vi "OscTest.vi"(7 "FrequencyCounter":refnum<visa-resource-name>, 8 "error in":errorcluster, 9 "connection information":path, 10 "System Number":string, 11 "Arduino":refnum<visa-resource-name>) -> (0 "error out":errorcluster, 3 "Arduino out":refnum<visa-resource-name>)   [LabVIEW 2024]
uses:
  <vilib>/addons/database/Connection.llb/DB Tools Open Connec (Path).vi
  Agilent 532XX Series/Public/Configure/Measurement/Configure Measurement (Frequency).vi
  <vilib>/addons/database/_DB Variant To Data/Database Variant To Data.xnode
  <vilib>/addons/database/NI_Database_API.lvlib
  Agilent 532XX Series/Agilent 532XX Series.lvlib
panel:
  out "Work Order":string
  out "Unit_Number":string
  out "VoltageSupply":dbl format="%.4f"
  out "Nominal Frequency":string
  out "IsSine":bool=TRUE
  out "TimeStart":string
  in  "DC_SN":string
  out "OscData":string
  out "VcLower":string
  out "VcLower-Frequency":dbl format="%.6f"
  out "Lower Deviation":dbl
  out "VcUpper":string
  out "VcUpper-Frequency":dbl format="%.6f"
  out "Upper Deviation":dbl
  out "VcMiddle-Frequency":dbl format="%.6f"
  out "Symmetry":dbl format="%.6f"
  out "State \"1\"":dbl format="%.6f"
  out "State \"0\"":dbl format="%.6f"
  out "Middle Deviation":dbl
  out "RiseTime":dbl format="%.6f"
  out "FallTime":dbl format="%.6f"
  out "Vpp":dbl format="%.6f"
  out "VcMiddle":string
  out "CurrentSupply":dbl format="%.4f"
  out "OscVoltage":string
types:
  T1 = typedef "NI_Database_API.lvlib/Conn ObjectReference.ctl" = refnum<k1>
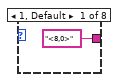
[diagram p3: hidden frame]
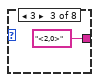
[diagram p4: hidden frame]
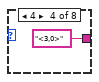
[diagram p5: hidden frame]
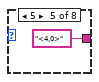
[diagram p6: hidden frame]
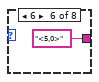
[diagram p7: hidden frame]
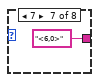
[diagram p8: hidden frame]
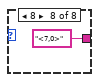
[diagram p9: hidden frame]
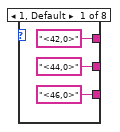
[diagram p10: hidden frame]
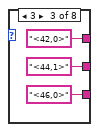
[diagram p11: hidden frame]
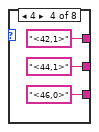
[diagram p12: hidden frame]
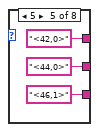
[diagram p13: hidden frame]
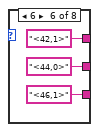
[diagram p14: hidden frame]
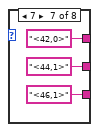
[diagram p15: hidden frame]
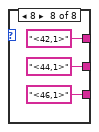
[diagram p16: hidden frame]
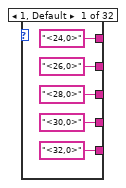
[diagram p17: hidden frame]
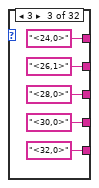
[diagram p18: hidden frame]
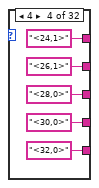
[diagram p19: hidden frame]
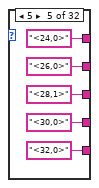
[diagram p20: hidden frame]
diagram:
  n1 = flat-sequence {
    tunnel: [w15] -> w1
    tunnel: w1 -> [w16]
    tunnel: [w23] -> w7
    tunnel: [w24] -> w6
    tunnel: w7 -> [w29]
    tunnel: w6 -> [w28]
    tunnel: [w27] -> w5
    tunnel: [w26] -> w4
    tunnel: [w862] -> w2
    tunnel: w5 -> [w862]
    tunnel: [w861] -> w3
    tunnel: w4 -> [w861]
    frame #0 {
      n2 = Get Date/Time In Seconds() -> (seconds since 1Jan1904=w14:timestamp)
      n3 = Bundle(0, 6) -> (w15:cluster{i32, i32})  [unwired: 1 in]
      n4 = Format Date/Time String(time format string (%c)="%m/%d/%Y %I:%M %p", seconds (now)=w14) -> (date/time string=→"TimeStart":string)  [unwired: 1 in]
      n5 = call "Set Temperature and Rise Time.vi"("Slew Time String"="0", "Temperature String"="25", "Device"=w15) -> ()  [unwired: 3 in, 1 out]
    }
    frame #1 {
      n6 = while {
        tunnel: w16 -> [w22]
        stop <- w18 stop-if-true
        n7 = call "Read Saunders Temperature.vi"("Device"=w22) -> ("Temperature"=w21:dbl)  [unwired: 3 in, 1 out]
        n8 = Wait (ms)(milliseconds to wait=u32 1000) -> ()  [unwired: 1 out]
        n9 = In Range and Coerce(upper limit=26.0, x=w21, lower limit=24.0) -> (In Range?=w18:bool)  [unwired: 1 out]
      }
    }
    frame #2 {
      n10 = local read "Arduino"() -> (w23:refnum<visa-resource-name>)
      n11 = local read "error in"() -> (w24:errorcluster)
      n12 = Wait (ms)(milliseconds to wait=u32 500) -> ()  [unwired: 1 out]
    }
    frame #3 {
      n13 = for {
        N: 32 -> [_]
        shift-right: [w32] -> w27
        shift-left: w29 -> [w34]
        shift-right: [w31] -> w26
        shift-left: w28 -> [w33]
        i -> [w35]
        n14 = for {
          N: 8 -> [_]
          tunnel: w35 -> [w47]
          shift-right: [w44] -> w32
          shift-left: w34 -> [w46]
          shift-right: [w43] -> w31
          shift-left: w33 -> [w45]
          i -> [w49]
          n15 = Increment(x=w49) -> (x+1=w48:i32)
          n16 = flat-sequence {
            tunnel: [w53] -> w42
            tunnel: [w84] -> w41
            tunnel: [w83] -> w40
            tunnel: [w82] -> w39
            tunnel: w48 -> [w53]
            tunnel: w47 -> [w50]
            tunnel: w46 -> [w83]
            tunnel: w45 -> [w80]
            tunnel: [w52] -> w38
            tunnel: [w51] -> w37
            tunnel: w42 -> [w137]
            tunnel: w41 -> [w136]
            tunnel: w40 -> [w135]
            tunnel: w39 -> [w134]
            tunnel: [w133] -> w44
            tunnel: [w132] -> w43
            tunnel: w38 -> [w131]
            tunnel: w37 -> [w130]
            frame #0 {
              n17 = local read "System Number"() -> (w68:string)
              n18 = local write "DC_SN"("" ("DC.SN")) -> ()
              n19 = local read "connection information"() -> (w54:path)
              n20 = Number To Decimal String(number=w53) -> (decimal integer string=w69:string)  [unwired: 1 in]
              n21 = Concatenate Strings("WHERE System=" ("SQL Query"), w68, " AND Rack=", w69, ";" ("string")) -> (w55:string)
              n22 = call-poly <vilib>:"DB Tools Open Connection.vi"("connection information"=w54) -> ("error out"=w65:errorcluster, "connection reference"=w66:T1)  [unwired: 7 in]
              n23 = Increment(x=w50) -> (x+1=w84:i32)
              n24 = call <vilib>:"DB Tools Select Data.vi"("condition"=w55, "error in (no error)"=w65, "columns"=string[] ["Position"], "table"="ACTIVE", "connection reference"=w66) -> ("error out"=w62:errorcluster, "data"=w60:variant[][], "connection reference out"=w64:T1)  [unwired: 1 in]
              n25 = xnode "Database Variant To Data"("database variant"=w60, "error in (no error)"=w62, "type"=string[][] [] ("DC.SN")) -> ("data"=w59:string[][], "error out"=w63:errorcluster)
              n26 = call <vilib>:"DB Tools Close Connection.vi"("error in (no error)"=w63, "connection reference"=w64) -> ("error out"=w56:errorcluster)  [unwired: 5 in]
              n27 = Index Array(array=w59, index (row)=0 ("disabled index (row)"), index (col)=0 ("disabled index (col)")) -> (element=w79:string)
              n28 = Unbundle By Name(w56) -> ("status"=w67:bool)
              n29 = call <vilib>:"Delimited String to 1D String Array.vi"("delimiter"=",", "delimited string"=w79) -> ("string array"=w76:string[])  [unwired: 9 in]
              n30 = Not(x=w67) -> (.not. x?=w52:bool)
              n31 = Index Array(array=w76, index=w50) -> (element=w75:string)
              n32 = call <vilib>:"Clear Errors.vi"("error in (no error)"=w80) -> ("error out"=w82:errorcluster)  [unwired: 5 in, 1 out]
              n33 = Equal?(x="1", y=w75) -> (x = y?=w51:bool)
            }
            frame #1 {
              n34 = And(x=w130, y=w131) -> (x .and. y?=w129:bool)
              n35 = case shown="True" w129 {
                tunnel: w136 -> [_ w183]
                tunnel: w137 -> [_ w182]
                tunnel: w135 -> [w138 w172]
                tunnel: w134 -> [w139 w173]
                tunnel: [w138 w160] -> w133
                tunnel: [w139 w159] -> w132
                frame False {
                }
                frame True {
                  n36 = flat-sequence {
                    tunnel: w182 -> [w189]
                    tunnel: w183 -> [w190]
                    tunnel: [w190] -> w180
                    tunnel: [w189] -> w178
                    tunnel: [w184] -> w142
                    tunnel: w180 -> [w394]
                    tunnel: [w394] -> w179
                    tunnel: w178 -> [w393]
                    tunnel: [w393] -> w177
                    tunnel: [w391] -> w143
                    tunnel: w142 -> [w391]
                    tunnel: [w400] -> w175
                    tunnel: w179 -> [w397]
                    tunnel: w177 -> [w400]
                    tunnel: [w438] -> w144
                    tunnel: w143 -> [w438]
                    tunnel: [w395] -> w141
                    tunnel: w175 -> [w486]
                    tunnel: [w486] -> w174
                    tunnel: [w484] -> w145
                    tunnel: w144 -> [w484]
                    tunnel: w141 -> [w483]
                    tunnel: [w483] -> w140
                    tunnel: w174 -> [w493]
                    tunnel: [w493] -> w176
                    tunnel: w173 -> [w492]
                    tunnel: w172 -> [w491]
                    tunnel: [w489] -> w170
                    tunnel: [w490] -> w169
                    tunnel: w145 -> [w488]
                    tunnel: w140 -> [w487]
                    tunnel: w176 -> [w501]
                    tunnel: [w501] -> w181
                    tunnel: w181 -> [w512]
                    tunnel: [w512] -> w168
                    tunnel: [w503] -> w165
                    tunnel: w168 -> [w515]
                    tunnel: [w515] -> w167
                    tunnel: [w513] -> w166
                    tunnel: w165 -> [w513]
                    tunnel: w167 -> [w516]
                    tunnel: [w516] -> w171
                    tunnel: w166 -> [w520]
                    tunnel: [w517] -> w162
                    tunnel: [w526] -> w164
                    tunnel: w171 -> [w526]
                    tunnel: [w524] -> w163
                    tunnel: w162 -> [w524]
                    tunnel: w164 -> [w537]
                    tunnel: [w537] -> w161
                    tunnel: w163 -> [w530]
                    tunnel: [w540] -> w158
                    tunnel: w161 -> [w539]
                    tunnel: [w539] -> w153
                    tunnel: w170 -> [w555]
                    tunnel: w169 -> [w554]
                    tunnel: [w553] -> w152
                    tunnel: [w552] -> w150
                    tunnel: w158 -> [w551]
                    tunnel: [w550] -> w154
                    tunnel: w153 -> [w550]
                    tunnel: [w556] -> w155
                    tunnel: w154 -> [w556]
                    tunnel: [w558] -> w156
                    tunnel: w155 -> [w558]
                    tunnel: [w574] -> w157
                    tunnel: w156 -> [w574]
                    tunnel: w157 -> [w576]
                    tunnel: w152 -> [w580]
                    tunnel: [w579] -> w151
                    tunnel: w150 -> [w578]
                    tunnel: [w577] -> w149
                    tunnel: [w576] -> w146
                    tunnel: [w840] -> w147
                    tunnel: w146 -> [w840]
                    tunnel: [w843] -> w148
                    tunnel: w147 -> [w843]
                    tunnel: w149 -> [w851]
                    tunnel: [w850] -> w160
                    tunnel: w151 -> [w849]
                    tunnel: [w848] -> w159
                    tunnel: w148 -> [w845]
                    frame #0 {
                      n37 = case shown="2" w189 {
                        tunnel: ["<8,0>" ("string") "<9,0>" ("string") "<2,0>" ("string") "<3,0>" ("string") "<4,0>" ("string") "<5,0>" ("string") "<6,0>" ("string") "<7,0>" ("string")] -> w188
                        frame 1, Default {
                        }
                        frame 2 {
                        }
                        frame 3 {
                        }
                        frame 4 {
                        }
                        frame 5 {
                        }
                        frame 6 {
                        }
                        frame 7 {
                        }
                        frame 8 {
                        }
                      }
                      n38 = case shown="2" w189 {
                        tunnel: ["<42,0>" ("string") "<42,1>" ("string") "<42,0>" ("string") "<42,1>" ("string") "<42,0>" ("string") "<42,1>" ("string") "<42,0>" ("string") "<42,1>" ("string")] -> w193
                        tunnel: ["<44,0>" ("string") "<44,0>" ("string") "<44,1>" ("string") "<44,1>" ("string") "<44,0>" ("string") "<44,0>" ("string") "<44,1>" ("string") "<44,1>" ("string")] -> w192
                        tunnel: ["<46,0>" ("string") "<46,0>" ("string") "<46,0>" ("string") "<46,0>" ("string") "<46,1>" ("string") "<46,1>" ("string") "<46,1>" ("string") "<46,1>" ("string")] -> w191
                        frame 1, Default {
                        }
                        frame 2 {
                        }
                        frame 3 {
                        }
                        frame 4 {
                        }
                        frame 5 {
                        }
                        frame 6 {
                        }
                        frame 7 {
                        }
                        frame 8 {
                        }
                      }
                      n39 = case shown="2" w190 {
                        tunnel: ["<32,0>" ("string") "<32,0>" ("string") "<32,0>" ("string") "<32,0>" ("string") "<32,0>" ("string") "<32,0>" ("string") "<32,0>" ("string") "<32,0>" ("string") "<32,0>" ("string") "<32,0>" ("string") "<32,0>" ("string") "<32,0>" ("string") "<32,0>" ("string") "<32,0>" ("string") "<32,0>" ("string") "<32,0>" ("string") "<32,1>" ("string") "<32,1>" ("string") "<32,1>" ("string") "<32,1>" ("string") "<32,1>" ("string") "<32,1>" ("string") "<32,1>" ("string") "<32,1>" ("string") "<32,1>" ("string") "<32,1>" ("string") "<32,1>" ("string") "<32,1>" ("string") "<32,1>" ("string") "<32,1>" ("string") "<32,1>" ("string") "<32,1>" ("string")] -> w194
                        tunnel: ["<30,0>" ("string") "<30,0>" ("string") "<30,0>" ("string") "<30,0>" ("string") "<30,0>" ("string") "<30,0>" ("string") "<30,0>" ("string") "<30,0>" ("string") "<30,1>" ("string") "<30,1>" ("string") "<30,1>" ("string") "<30,1>" ("string") "<30,1>" ("string") "<30,1>" ("string") "<30,1>" ("string") "<30,1>" ("string") "<30,0>" ("string") "<30,0>" ("string") "<30,0>" ("string") "<30,0>" ("string") "<30,0>" ("string") "<30,0>" ("string") "<30,0>" ("string") "<30,0>" ("string") "<30,1>" ("string") "<30,1>" ("string") "<30,1>" ("string") "<30,1>" ("string") "<30,1>" ("string") "<30,1>" ("string") "<30,1>" ("string") "<30,1>" ("string")] -> w195
                        tunnel: ["<28,0>" ("string") "<28,0>" ("string") "<28,0>" ("string") "<28,0>" ("string") "<28,1>" ("string") "<28,1>" ("string") "<28,1>" ("string") "<28,1>" ("string") "<28,0>" ("string") "<28,0>" ("string") "<28,0>" ("string") "<28,0>" ("string") "<28,1>" ("string") "<28,1>" ("string") "<28,1>" ("string") "<28,1>" ("string") "<28,0>" ("string") "<28,0>" ("string") "<28,0>" ("string") "<28,0>" ("string") "<28,1>" ("string") "<28,1>" ("string") "<28,1>" ("string") "<28,1>" ("string") "<28,0>" ("string") "<28,0>" ("string") "<28,0>" ("string") "<28,0>" ("string") "<28,1>" ("string") "<28,1>" ("string") "<28,1>" ("string") "<28,1>" ("string")] -> w196
                        tunnel: ["<26,0>" ("string") "<26,0>" ("string") "<26,1>" ("string") "<26,1>" ("string") "<26,0>" ("string") "<26,0>" ("string") "<26,1>" ("string") "<26,1>" ("string") "<26,0>" ("string") "<26,0>" ("string") "<26,1>" ("string") "<26,1>" ("string") "<26,0>" ("string") "<26,0>" ("string") "<26,1>" ("string") "<26,1>" ("string") "<26,0>" ("string") "<26,0>" ("string") "<26,1>" ("string") "<26,1>" ("string") "<26,0>" ("string") "<26,0>" ("string") "<26,1>" ("string") "<26,1>" ("string") "<26,0>" ("string") "<26,0>" ("string") "<26,1>" ("string") "<26,1>" ("string") "<26,0>" ("string") "<26,0>" ("string") "<26,1>" ("string") "<26,1>" ("string")] -> w197
                        tunnel: ["<24,0>" ("string") "<24,1>" ("string") "<24,0>" ("string") "<24,1>" ("string") "<24,0>" ("string") "<24,1>" ("string") "<24,0>" ("string") "<24,1>" ("string") "<24,0>" ("string") "<24,1>" ("string") "<24,0>" ("string") "<24,1>" ("string") "<24,0>" ("string") "<24,1>" ("string") "<24,0>" ("string") "<24,1>" ("string") "<24,0>" ("string") "<24,1>" ("string") "<24,0>" ("string") "<24,1>" ("string") "<24,0>" ("string") "<24,1>" ("string") "<24,0>" ("string") "<24,1>" ("string") "<24,0>" ("string") "<24,1>" ("string") "<24,0>" ("string") "<24,1>" ("string") "<24,0>" ("string") "<24,1>" ("string") "<24,0>" ("string") "<24,1>" ("string")] -> w198
                        frame 1, Default {
                        }
                        frame 2 {
                        }
                        frame 3 {
                        }
                        frame 4 {
                        }
                        frame 5 {
                        }
                        frame 6 {
                        }
                        frame 7 {
                        }
                        frame 8 {
                        }
                        frame 9 {
                        }
                        frame 10 {
                        }
                        frame 11 {
                        }
                        frame 12 {
                        }
                        frame 13 {
                        }
                        frame 14 {
                        }
                        frame 15 {
                        }
                        frame 16 {
                        }
                        frame 17 {
                        }
                        frame 18 {
                        }
                        frame 19 {
                        }
                        frame 20 {
                        }
                        frame 21 {
                        }
                        frame 22 {
                        }
                        frame 23 {
                        }
                        frame 24 {
                        }
                        frame 25 {
                        }
                        frame 26 {
                        }
                        frame 27 {
                        }
                        frame 28 {
                        }
                        frame 29 {
                        }
                        frame 30 {
                        }
                        frame 31 {
                        }
                        frame 32 {
                        }
                      }
                      n40 = Build Array(w188, w193, w192, w191, w198, w197, w196, w195, w194, "<48,0>" ("string"), "<50,0>" ("string"), "<52,0>" ("string")) -> (w184:string[])
                    }
                    frame #1 {
                      n41 = Wait (ms)(milliseconds to wait=u32 500) -> ()  [unwired: 1 out]
                    }
                    frame #2 {
                      # "Gets the latest TimeStart from this System/Rack/Position meaning it will be associated with the oscillator that is currently in the spot"
                      # "Data Grabbed:\nIsSine:\n-Boolean that identifies if the Waveform is equal to sine to ensure the frequency counter can be set up for the correct wave\nOscVoltage:\n-The amount of voltage that the oscillator receives as input\nGate Time \n-The period over which the counter accumulates the number of input signal cycles\nNominal Frequency\n- Reference value or a standard against which other frequencies are measured or compared\nDC_SN\n-Unique date code/serial number that identifies the device that is being tested"
                      # "Gets the latest TimeStart from this System/Rack/Position meaning it will be associated with the oscillator that is currently in the spot"
                      n42 = local read "connection information"() -> (w407:path)
                      n43 = local read "System Number"() -> (w437:string)
                      n44 = Number To Decimal String(number=w400) -> (decimal integer string=w403:string)  [unwired: 1 in]
                      n45 = Number To Decimal String(number=w397) -> (decimal integer string=w396:string)  [unwired: 1 in]
                      n46 = Concatenate Strings("WHERE SystemNumber=" ("SQL Query"), w437, "AND RackNumber=" ("string"), w403, "AND PositionNumber=" ("string"), w396, "ORDER BY TimeStart DESC" ("string")) -> (w406:string)
                      n47 = call-poly <vilib>:"DB Tools Open Connection.vi"("connection information"=w407) -> ("error out"=w414:errorcluster, "connection reference"=w415:T1)  [unwired: 7 in]
                      n48 = call <vilib>:"DB Tools Select Data.vi"("condition"=w406, "error in (no error)"=w414, "table"="MASTER", "connection reference"=w415) -> ("error out"=w411:errorcluster, "data"=w409:variant[][], "connection reference out"=w413:T1)  [unwired: 2 in]
                      n49 = xnode "Database Variant To Data"("database variant"=w409, "error in (no error)"=w411, "type"=string[][] [] ("DC.SN")) -> ("data"=w405:string[][], "error out"=w412:errorcluster)
                      n50 = call <vilib>:"DB Tools Close Connection.vi"("error in (no error)"=w412, "connection reference"=w413) -> ("error out"=w404:errorcluster)  [unwired: 5 in]
                      n51 = Index Array(array=w405, index (row)=0 ("disabled index (row)")) -> (element=w419:string[])  [unwired: 1 in]
                      n52 = Unbundle By Name(w404) -> ("status"=w424:bool)
                      n53 = Index Array(array=w419, index=8) -> (element=w430:string)
                      n54 = Index Array(array=w419, index=0) -> (element=w429:string)
                      n55 = Index Array(array=w419, index=9) -> (element=→"OscVoltage":string)
                      n56 = Index Array(array=w419, index=1) -> (element=w418:string)
                      n57 = Index Array(array=w419, index=2) -> (element=w416:string)
                      n58 = Index Array(array=w419, index=12) -> (element=w402:string)
                      n59 = Index Array(array=w419, index=10) -> (element=w431:string)
                      n60 = local write "Nominal Frequency"(w430) -> ()
                      n61 = local write "DC_SN"(w429) -> ()
                      n62 = local write "Unit_Number"(w402) -> ()
                      n63 = Concatenate Strings(w418, "-" ("string"), w416) -> (w401:string)
                      n64 = Equal?(x="Sine", y=w431) -> (x = y?=w398:bool)
                      n65 = local write "Work Order"(w401) -> ()
                      n66 = local write "IsSine"(w398) -> ()
                      n67 = Not(x=w424) -> (.not. x?=w395:bool)
                    }
                    frame #3 {
                      n68 = Wait (ms)(milliseconds to wait=u32 500) -> ()  [unwired: 1 out]
                    }
                    frame #4 {
                      n69 = case shown="True" w487 {
                        tunnel: w492 -> [w495 w500]
                        tunnel: w491 -> [w494 w499]
                        tunnel: [w494 w498] -> w490
                        tunnel: [w495 w497] -> w489
                        tunnel: w488 -> [_ w496]
                        frame False {
                        }
                        frame True {
                          n70 = call "Arduino Command Builder.vi"("error in"=w500, "Commands"=w496, "Arduino in"=w499) -> ("error out"=w497:errorcluster, "Arduino out"=w498:refnum<visa-resource-name>)  [unwired: 7 in]
                        }
                      }
                    }
                    frame #5 {
                      n71 = Wait (ms)(milliseconds to wait=u32 1000 ("millisecond multiple")) -> ()  [unwired: 1 out]
                    }
                    frame #6 {
                      w508 = u16 0 items=["channel 1", "channel 2", "channel 3"] ("channel (ch1:0)")
                      # "Sets the current and voltage limits, and ensures they are within a range to prevent anything from blowing up for channel 1"
                      # "Sets the voltage equal to the value of the OscVoltage which is gotten from the part number (channel 1)"
                      n72 = local read "OscVoltage"() -> (w511:string)
                      n73 = Fract/Exp String To Number(string=w511) -> (number=w504:dbl)  [unwired: 3 in, 1 out]
                      n74 = call "Tek PS2520G Configure Supply24.vi"("GPIB #"=u8 0, "voltage limit"=w504, "Address"=u8 8, "channel (ch1:0)"=w508, "current limit"=1.5, "Switch Output"=TRUE, "output (t:on)"=TRUE) -> ("error out"=w503:errorcluster)  [unwired: 1 in]
                    }
                    frame #7 {
                      n75 = Wait (ms)(milliseconds to wait=u32 1000) -> ()  [unwired: 1 out]
                    }
                    frame #8 {
                      w521 = u16 0 items=["channel 1", "channel 2", "channel 3"] ("channel (ch1:0)")
                      n76 = call "Tek PS2520G Check Volt and Current24.vi"("GPIB #"=u8 0, "Address"=u8 8, "channel (ch1:0)"=w521, "error in (no error)"=w520) -> ("actual output voltage"=→"VoltageSupply":dbl, "actual output current"=→"CurrentSupply":dbl, "error out"=w517:errorcluster)  [unwired: 2 in]
                    }
                    frame #9 {
                      n77 = Wait (ms)(milliseconds to wait=u32 1000) -> ()  [unwired: 1 out]
                    }
                    frame #10 {
                      w532 = u16 0 items=["channel 1", "channel 2", "channel 3"] ("channel (ch1:0)")
                      n78 = call "Tek PS2520G Configure Supply24.vi"("GPIB #"=u8 0, "voltage limit"=0.0, "Address"=u8 8, "channel (ch1:0)"=w532, "current limit"=1.5, "error in (no error)"=w530, "Switch Output"=FALSE, "output (t:on)"=FALSE) -> ("error out"=w527:errorcluster)
                      n79 = Unbundle By Name(w527) -> ("status"=w536:bool)
                      n80 = case shown="False" w536 {
                        frame False {
                        }
                        frame True {
                          n81 = VISA Clear(VISA resource name=refnum<visa-resource-name> "GPIB0::8::INSTR") -> ()  [unwired: 1 in, 2 out]
                        }
                      }
                    }
                    frame #11 {
                      n82 = case shown="2" w539 {
                        tunnel: ["<8,1>" ("string") "<9,1>" ("string") "<2,1>" ("string") "<3,1>" ("string") "<4,1>" ("string") "<5,1>" ("string") "<6,1>" ("string") "<7,1>" ("string")] -> w541
                        frame 1, Default {
                        }
                        frame 2 {
                        }
                        frame 3 {
                        }
                        frame 4 {
                        }
                        frame 5 {
                        }
                        frame 6 {
                        }
                        frame 7 {
                        }
                        frame 8 {
                        }
                      }
                      n83 = Build Array(w541) -> (w540:string[])
                    }
                    frame #12 {
                      n84 = call "Arduino Command Builder.vi"("error in"=w555, "Commands"=w551, "Arduino in"=w554) -> ("error out"=w553:errorcluster, "Arduino out"=w552:refnum<visa-resource-name>)  [unwired: 7 in]
                    }
                    frame #13 {
                      n85 = Wait (ms)(milliseconds to wait=u32 500 ("millisecond multiple")) -> ()  [unwired: 1 out]
                    }
                    frame #14 {
                      n86 = disable-structure shown="Enabled" {
                        frame Disabled {
                          # "Setting the Impedance and Coupling for AC or DC"
                          n87 = local read "IsSine"() -> (w559:bool)
                          n88 = case shown="True" w559 {
                            frame False {
                              n89 = flat-sequence {
                                frame #0 {
                                n90 = Send(0:0 ("bus"), 2:i16 3 ("address"), 5:"INP:COUP DC " ("data string")) -> ()  [unwired: 2 in, 3 out]
                                }
                                frame #1 {
                                n91 = Wait (ms)(milliseconds to wait=u32 500 ("millisecond multiple")) -> ()  [unwired: 1 out]
                                }
                                frame #2 {
                                n92 = Send(0:0 ("bus"), 2:i16 3 ("address"), 5:"INP:IMP 1.0E6" ("data string")) -> ()  [unwired: 2 in, 3 out]
                                }
                              }
                            }
                            frame True {
                              n93 = flat-sequence {
                                frame #0 {
                                n94 = Send(0:0 ("bus"), 2:i16 3 ("address"), 5:"INP:COUP AC " ("data string")) -> ()  [unwired: 2 in, 3 out]
                                }
                                frame #1 {
                                n95 = Wait (ms)(milliseconds to wait=u32 500 ("millisecond multiple")) -> ()  [unwired: 1 out]
                                }
                                frame #2 {
                                n96 = Send(0:0 ("bus"), 2:i16 3 ("address"), 5:"INP:IMP 50" ("data string")) -> ()  [unwired: 2 in, 3 out]
                                }
                              }
                            }
                          }
                        }
                        frame Enabled {
                        }
                      }
                    }
                    frame #15 {
                      n97 = Wait (ms)(milliseconds to wait=u32 500 ("millisecond multiple")) -> ()  [unwired: 1 out]
                    }
                    frame #16 {
                      n98 = flat-sequence {
                        tunnel: w576 -> [w621]
                        tunnel: [w619] -> w581
                        tunnel: w581 -> [w634]
                        tunnel: w580 -> [w633]
                        tunnel: [w632] -> w579
                        tunnel: w578 -> [w630]
                        tunnel: [w631] -> w577
                        frame #0 {
                          w582 = 0.0 ("Is")
                          # "Resets all these variables"
                          n99 = local write "State \"0\""(w582) -> ()
                          n100 = local write "FallTime"(w582) -> ()
                          n101 = local write "VcMiddle-Frequency"(w582) -> ()
                          n102 = local write "VcUpper-Frequency"(w582) -> ()
                          n103 = local write "Symmetry"(w582) -> ()
                          n104 = local write "VcLower-Frequency"(w582) -> ()
                          n105 = local write "State \"1\""(w582) -> ()
                          n106 = local write "RiseTime"(w582) -> ()
                        }
                        frame #1 {
                          n107 = Wait (ms)(milliseconds to wait=u32 500 ("millisecond multiple")) -> ()  [unwired: 1 out]
                          n108 = VISA Clear(VISA resource name=refnum<visa-resource-name> "GPIB0::3::INSTR") -> ()  [unwired: 1 in, 2 out]
                        }
                        frame #2 {
                          # "Grabs all the relevant data for the wave at its true voltage and the current that it draws from it"
                          # "Grabs the Frequency and accounts for error values that are out of range based on nominal frequency"
                          n109 = call "Frequency Counter Waveform.vi"("Channel(1,2,3)"=enum16{"Channel 1", "Channel 2", "Channel 3"}."Channel 1", "VISA resource name"=refnum<visa-resource-name> "GPIB0::3::INSTR") -> ("Symmetry"=→"Symmetry":dbl, "Vmax"=w604:dbl, "Vmin"=w605:dbl, "RTime"=w608:dbl, "FTime"=w607:dbl, "error out"=w592:errorcluster)  [unwired: 7 in, 1 out]
                          n110 = Unbundle By Name(w592) -> ("status"=w591:bool)
                          n111 = In Range and Coerce(upper limit=20.0, x=w604, lower limit=-20.0) -> (coerced(x)=w589:dbl)  [unwired: 1 out]
                          n112 = In Range and Coerce(upper limit=20.0, x=w605, lower limit=-20.0) -> (coerced(x)=w587:dbl)  [unwired: 1 out]
                          n113 = In Range and Coerce(upper limit=500.0, x=w608, lower limit=0.0) -> (coerced(x)=→"RiseTime":dbl)  [unwired: 1 out]
                          n114 = In Range and Coerce(upper limit=500.0, x=w607, lower limit=0.0) -> (coerced(x)=→"FallTime":dbl)  [unwired: 1 out]
                          n115 = local read "IsSine"() -> (w590:bool)
                          n116 = case shown="True" w591 {
                            frame False {
                            }
                            frame True {
                              n117 = VISA Clear(VISA resource name=refnum<visa-resource-name> "GPIB0::3::INSTR") -> ()  [unwired: 1 in, 2 out]
                            }
                          }
                          n118 = case shown="True" w590 {
                            tunnel: w589 -> [w615 w617]
                            tunnel: [w611 w617] -> w588
                            tunnel: w587 -> [w614 w616]
                            tunnel: [w610 w616] -> w586
                            frame False {
                              n119 = Divide(x=w615, y=0.185) -> (x/y=w611:dbl)
                              n120 = Divide(x=w614, y=0.185) -> (x/y=w610:dbl)
                            }
                            frame True {
                            }
                          }
                          "State \"1\"" <- w588
                          "State \"0\"" <- w586
                          n121 = Subtract(x=w589, y=w587) -> (x-y=→"Vpp":dbl)
                        }
                        frame #3 {
                          n122 = case shown="1, Default" w621 {
                            tunnel: ["<21,1>" ("string") "<20,1>" ("string") "<19,1>" ("string") "<18,1>" ("string") "<17,1>" ("string") "<16,1>" ("string") "<15,1>" ("string") "<14,1>" ("string")] -> w620
                            frame 1, Default {
                            }
                            frame 2 {
                            }
                            frame 3 {
                            }
                            frame 4 {
                            }
                            frame 5 {
                            }
                            frame 6 {
                            }
                            frame 7 {
                            }
                            frame 8 {
                            }
                          }
                          n123 = Build Array(w620) -> (w619:string[])
                        }
                        frame #4 {
                          n124 = call "Arduino Command Builder.vi"("error in"=w633, "Commands"=w634, "Arduino in"=w630) -> ("error out"=w632:errorcluster, "Arduino out"=w631:refnum<visa-resource-name>)  [unwired: 7 in]
                        }
                        frame #5 {
                          n125 = Wait (ms)(milliseconds to wait=u32 1000) -> ()  [unwired: 1 out]
                        }
                        frame #6 {
                          n126 = flat-sequence {
                            tunnel: [w655] -> w639
                            tunnel: [w662] -> w638
                            tunnel: w639 -> [w662]
                            tunnel: w638 -> [w665]
                            tunnel: [w664] -> w636
                            tunnel: [w676] -> w637
                            frame #0 {
                              w659 = u16 1 items=["channel 1", "channel 2", "channel 3"] ("channel (ch1:0)")
                              n127 = local read "OscVoltage"() -> (w652:string)
                              n128 = Format Value(string ("")=w652, format string="%.2p") -> (output string=w651:string)  [unwired: 1 in]
                              n129 = Fract/Exp String To Number(use system decimal point (T)=TRUE, string=w651, default (0 dbl)=0.0 ("default (0 DBL)")) -> (number=w648:dbl)  [unwired: 1 in, 1 out]
                              n130 = Divide(x=w648, y=2.0) -> (x/y=w647:dbl)
                              n131 = call "Tek PS2520G Configure Supply24.vi"("GPIB #"=u8 0, "voltage limit"=w647, "Address"=u8 8, "channel (ch1:0)"=w659, "current limit"=1.5, "Switch Output"=FALSE, "output (t:on)"=TRUE) -> ("error out"=w655:errorcluster)  [unwired: 1 in]
                            }
                            frame #1 {
                              n132 = Wait (ms)(milliseconds to wait=u32 5000) -> ()  [unwired: 1 out]
                            }
                            frame #2 {
                              w666 = u16 1 items=["channel 1", "channel 2", "channel 3"] ("channel (ch1:0)")
                              n133 = call "Tek PS2520G Check Volt and Current24.vi"("GPIB #"=u8 0, "Address"=u8 8, "channel (ch1:0)"=w666, "error in (no error)"=w665) -> ("actual output voltage"=w670:dbl, "error out"=w669:errorcluster)  [unwired: 2 in, 1 out]
                              n134 = Unbundle By Name(w669) -> ("status"=w671:bool)
                              n135 = Number To Fractional String(number=w670, precision (6)=i16 2) -> (F-format string=w664:string)  [unwired: 2 in]
                              n136 = case shown="False" w671 {
                                frame False {
                                }
                                frame True {
                                n137 = VISA Clear(VISA resource name=refnum<visa-resource-name> "GPIB0::8::INSTR") -> ()  [unwired: 1 in, 2 out]
                                }
                              }
                            }
                            frame #3 {
                              n138 = Wait (ms)(milliseconds to wait=u32 500) -> ()  [unwired: 1 out]
                            }
                            frame #4 {
                              n139 = for {
                                N: 5 -> [_]
                                tunnel: [w677] -> w676
                                stop <- w678 continue-if-true
                                w682 = 1 items=["Channel 1"=1, "Channel 2"=2, "Channel 3"=3] ("Channel (1:Channel 1)")
                                n140 = local read "FrequencyCounter"() -> (w689:refnum<visa-resource-name>)
                                n141 = call "Initialize.vi"("VISA resource name"=w689) -> ("error out"=w684:errorcluster, "VISA resource name out"=w683:refnum<visa-resource-name>)  [unwired: 9 in]
                                n142 = call "Configure Frequency Gate.vi"("error in (no error)"=w684, "Time Resolution (0.1 s)"=0.1 ("number"), "VISA resource name"=w683) -> ("error out"=w693:errorcluster, "VISA resource name out"=w690:refnum<visa-resource-name>)  [unwired: 7 in]
                                n143 = call-poly "Configure Measurement.vi"("error in (no error)"=w693, "Channel (1:Channel 1)"=w682, "VISA resource name"=w690) -> ("error out"=w692:errorcluster, "VISA resource name out"=w691:refnum<visa-resource-name>)  [unwired: 2 in, 5 out]
                                n144 = call "Read Measurement (Single).vi"("error in (no error)"=w692, "VISA resource name"=w691) -> ("error out"=w686:errorcluster, "Measurement"=w687:dbl, "VISA resource name out"=w685:refnum<visa-resource-name>)  [unwired: 7 in]
                                n145 = call "Close.vi"("error in (no error)"=w686, "VISA resource name"=w685) -> ("error out"=w688:errorcluster)  [unwired: 9 in]
                                n146 = In Range and Coerce(upper limit=5000000000.0, x=w687, lower limit=0.0) -> (coerced(x)=w677:dbl)  [unwired: 1 out]
                                n147 = Unbundle By Name(w688) -> ("status"=w678:bool)
                                n148 = case shown="True" w678 {
                                frame False {
                                }
                                frame True {
                                n149 = local read "FrequencyCounter"() -> (w694:refnum<visa-resource-name>)
                                n150 = VISA Clear(VISA resource name=w694) -> ()  [unwired: 1 in, 2 out]
                                }
                                }
                              }
                            }
                          }
                          n151 = local read "Nominal Frequency"() -> (w645:string)
                          n152 = Fract/Exp String To Number(string=w645) -> (number=w646:dbl)  [unwired: 3 in, 1 out]
                          n153 = Multiply(x=w646, y=1000000.0) -> (x*y=w644:dbl)
                          n154 = Subtract(x=w637, y=w644) -> (x-y=w642:dbl)
                          n155 = Absolute Value(x=w642) -> (abs(x)=w641:dbl)
                          n156 = Divide(x=w641, y=w646) -> (x/y=→"Middle Deviation":dbl)
                          "VcMiddle-Frequency" <- w637
                          "VcMiddle" <- w636
                        }
                        frame #7 {
                          n157 = Wait (ms)(milliseconds to wait=u32 1000) -> ()  [unwired: 1 out]
                        }
                        frame #8 {
                          n158 = flat-sequence {
                            tunnel: [w712] -> w701
                            tunnel: [w719] -> w702
                            tunnel: w701 -> [w719]
                            tunnel: w702 -> [w722]
                            tunnel: [w733] -> w704
                            frame #0 {
                              w716 = u16 1 items=["channel 1", "channel 2", "channel 3"] ("channel (ch1:0)")
                              n159 = local read "OscVoltage"() -> (w708:string)
                              n160 = Format Value(string ("")=w708, format string="%.2p") -> (output string=w707:string)  [unwired: 1 in]
                              n161 = Fract/Exp String To Number(use system decimal point (T)=TRUE, string=w707, default (0 dbl)=0.0 ("default (0 DBL)")) -> (number=w711:dbl)  [unwired: 1 in, 1 out]
                              n162 = call "Tek PS2520G Configure Supply24.vi"("GPIB #"=u8 0, "voltage limit"=w711, "Address"=u8 8, "channel (ch1:0)"=w716, "current limit"=1.5, "Switch Output"=FALSE, "output (t:on)"=TRUE) -> ("error out"=w712:errorcluster)  [unwired: 1 in]
                            }
                            frame #1 {
                              n163 = Wait (ms)(milliseconds to wait=u32 5000) -> ()  [unwired: 1 out]
                            }
                            frame #2 {
                              w723 = u16 1 items=["channel 1", "channel 2", "channel 3"] ("channel (ch1:0)")
                              n164 = call "Tek PS2520G Check Volt and Current24.vi"("GPIB #"=u8 0, "Address"=u8 8, "channel (ch1:0)"=w723, "error in (no error)"=w722) -> ("actual output voltage"=w727:dbl, "error out"=w726:errorcluster)  [unwired: 2 in, 1 out]
                              n165 = Unbundle By Name(w726) -> ("status"=w728:bool)
                              n166 = Number To Fractional String(number=w727, precision (6)=i16 2) -> (F-format string=→"VcUpper":string)  [unwired: 2 in]
                              n167 = case shown="True" w728 {
                                frame False {
                                }
                                frame True {
                                n168 = VISA Clear(VISA resource name=refnum<visa-resource-name> "GPIB0::8::INSTR") -> ()  [unwired: 1 in, 2 out]
                                }
                              }
                            }
                            frame #3 {
                              n169 = Wait (ms)(milliseconds to wait=u32 500) -> ()  [unwired: 1 out]
                            }
                            frame #4 {
                              n170 = for {
                                N: 5 -> [_]
                                tunnel: [w734] -> w733
                                stop <- w735 continue-if-true
                                w739 = 1 items=["Channel 1"=1, "Channel 2"=2, "Channel 3"=3] ("Channel (1:Channel 1)")
                                n171 = local read "FrequencyCounter"() -> (w746:refnum<visa-resource-name>)
                                n172 = call "Initialize.vi"("VISA resource name"=w746) -> ("error out"=w741:errorcluster, "VISA resource name out"=w740:refnum<visa-resource-name>)  [unwired: 9 in]
                                n173 = call "Configure Frequency Gate.vi"("error in (no error)"=w741, "Time Resolution (0.1 s)"=0.1 ("number"), "VISA resource name"=w740) -> ("error out"=w750:errorcluster, "VISA resource name out"=w747:refnum<visa-resource-name>)  [unwired: 7 in]
                                n174 = call-poly "Configure Measurement.vi"("error in (no error)"=w750, "Channel (1:Channel 1)"=w739, "VISA resource name"=w747) -> ("error out"=w749:errorcluster, "VISA resource name out"=w748:refnum<visa-resource-name>)  [unwired: 2 in, 5 out]
                                n175 = call "Read Measurement (Single).vi"("error in (no error)"=w749, "VISA resource name"=w748) -> ("error out"=w743:errorcluster, "Measurement"=w744:dbl, "VISA resource name out"=w742:refnum<visa-resource-name>)  [unwired: 7 in]
                                n176 = call "Close.vi"("error in (no error)"=w743, "VISA resource name"=w742) -> ("error out"=w745:errorcluster)  [unwired: 9 in]
                                n177 = In Range and Coerce(upper limit=5000000000.0, x=w744, lower limit=0.0) -> (coerced(x)=w734:dbl)  [unwired: 1 out]
                                n178 = Unbundle By Name(w745) -> ("status"=w735:bool)
                                n179 = case shown="False" w735 {
                                frame False {
                                }
                                frame True {
                                n180 = local read "FrequencyCounter"() -> (w751:refnum<visa-resource-name>)
                                n181 = VISA Clear(VISA resource name=w751) -> ()  [unwired: 1 in, 2 out]
                                }
                                }
                              }
                            }
                          }
                          n182 = local read "Nominal Frequency"() -> (w699:string)
                          n183 = Fract/Exp String To Number(string=w699) -> (number=w698:dbl)  [unwired: 3 in, 1 out]
                          n184 = Multiply(x=w698, y=1000000.0) -> (x*y=w700:dbl)
                          n185 = Subtract(x=w704, y=w700) -> (x-y=w697:dbl)
                          n186 = Absolute Value(x=w697) -> (abs(x)=w696:dbl)
                          n187 = Divide(x=w696, y=w698) -> (x/y=→"Upper Deviation":dbl)
                          "VcUpper-Frequency" <- w704
                        }
                        frame #9 {
                          n188 = Wait (ms)(milliseconds to wait=u32 1000) -> ()  [unwired: 1 out]
                        }
                        frame #10 {
                          n189 = flat-sequence {
                            tunnel: [w764] -> w759
                            tunnel: w759 -> [w772]
                            tunnel: [w772] -> w758
                            tunnel: w758 -> [w773]
                            tunnel: [w784] -> w761
                            frame #0 {
                              w768 = u16 1 items=["channel 1", "channel 2", "channel 3"] ("channel (ch1:0)")
                              n190 = call "Tek PS2520G Configure Supply24.vi"("GPIB #"=u8 0, "voltage limit"=0.0, "Address"=u8 8, "channel (ch1:0)"=w768, "current limit"=1.5, "Switch Output"=FALSE, "output (t:on)"=TRUE) -> ("error out"=w764:errorcluster)  [unwired: 1 in]
                            }
                            frame #1 {
                              n191 = Wait (ms)(milliseconds to wait=u32 5000) -> ()  [unwired: 1 out]
                            }
                            frame #2 {
                              w775 = u16 1 items=["channel 1", "channel 2", "channel 3"] ("channel (ch1:0)")
                              n192 = call "Tek PS2520G Check Volt and Current24.vi"("GPIB #"=u8 0, "Address"=u8 8, "channel (ch1:0)"=w775, "error in (no error)"=w773) -> ("actual output voltage"=w779:dbl, "error out"=w780:errorcluster)  [unwired: 2 in, 1 out]
                              n193 = Unbundle By Name(w780) -> ("status"=w778:bool)
                              n194 = Number To Fractional String(number=w779, precision (6)=i16 2) -> (F-format string=→"VcLower":string)  [unwired: 2 in]
                              n195 = case shown="True" w778 {
                                frame False {
                                }
                                frame True {
                                n196 = VISA Clear(VISA resource name=refnum<visa-resource-name> "GPIB0::8::INSTR") -> ()  [unwired: 1 in, 2 out]
                                }
                              }
                            }
                            frame #3 {
                              n197 = Wait (ms)(milliseconds to wait=u32 500) -> ()  [unwired: 1 out]
                            }
                            frame #4 {
                              n198 = for {
                                N: 5 -> [_]
                                tunnel: [w786] -> w784
                                stop <- w787 continue-if-true
                                w791 = 1 items=["Channel 1"=1, "Channel 2"=2, "Channel 3"=3] ("Channel (1:Channel 1)")
                                n199 = local read "FrequencyCounter"() -> (w798:refnum<visa-resource-name>)
                                n200 = call "Initialize.vi"("VISA resource name"=w798) -> ("error out"=w793:errorcluster, "VISA resource name out"=w792:refnum<visa-resource-name>)  [unwired: 9 in]
                                n201 = call "Configure Frequency Gate.vi"("error in (no error)"=w793, "Time Resolution (0.1 s)"=0.1 ("number"), "VISA resource name"=w792) -> ("error out"=w802:errorcluster, "VISA resource name out"=w799:refnum<visa-resource-name>)  [unwired: 7 in]
                                n202 = call-poly "Configure Measurement.vi"("error in (no error)"=w802, "Channel (1:Channel 1)"=w791, "VISA resource name"=w799) -> ("error out"=w801:errorcluster, "VISA resource name out"=w800:refnum<visa-resource-name>)  [unwired: 2 in, 5 out]
                                n203 = call "Read Measurement (Single).vi"("error in (no error)"=w801, "VISA resource name"=w800) -> ("error out"=w795:errorcluster, "Measurement"=w796:dbl, "VISA resource name out"=w794:refnum<visa-resource-name>)  [unwired: 7 in]
                                n204 = call "Close.vi"("error in (no error)"=w795, "VISA resource name"=w794) -> ("error out"=w797:errorcluster)  [unwired: 9 in]
                                n205 = In Range and Coerce(upper limit=5000000000.0, x=w796, lower limit=0.0) -> (coerced(x)=w786:dbl)  [unwired: 1 out]
                                n206 = Unbundle By Name(w797) -> ("status"=w787:bool)
                                n207 = case shown="False" w787 {
                                frame False {
                                }
                                frame True {
                                n208 = local read "FrequencyCounter"() -> (w803:refnum<visa-resource-name>)
                                n209 = VISA Clear(VISA resource name=w803) -> ()  [unwired: 1 in, 2 out]
                                }
                                }
                              }
                            }
                          }
                          n210 = local read "Nominal Frequency"() -> (w757:string)
                          n211 = Fract/Exp String To Number(string=w757) -> (number=w755:dbl)  [unwired: 3 in, 1 out]
                          n212 = Multiply(x=w755, y=1000000.0) -> (x*y=w756:dbl)
                          n213 = Subtract(x=w761, y=w756) -> (x-y=w754:dbl)
                          n214 = Absolute Value(x=w754) -> (abs(x)=w753:dbl)
                          n215 = Divide(x=w753, y=w755) -> (x/y=→"Lower Deviation":dbl)
                          "VcLower-Frequency" <- w761
                        }
                        frame #11 {
                          w805 = "," ("string")
                          # "Takes all the data recorded, and puts it into an array"
                          n216 = local read "Vpp"() -> (w813:dbl)
                          n217 = local read "VcMiddle-Frequency"() -> (w836:dbl)
                          n218 = local read "VcUpper-Frequency"() -> (w831:dbl)
                          n219 = local read "VcLower-Frequency"() -> (w829:dbl)
                          n220 = local read "Middle Deviation"() -> (w809:dbl)
                          n221 = local read "Upper Deviation"() -> (w826:dbl)
                          n222 = local read "Lower Deviation"() -> (w827:dbl)
                          n223 = local read "VoltageSupply"() -> (w806:dbl)
                          n224 = local read "CurrentSupply"() -> (w835:dbl)
                          n225 = Number To Fractional String(number=w813) -> (F-format string=w811:string)  [unwired: 3 in]
                          n226 = local read "Symmetry"() -> (w814:dbl)
                          n227 = local read "RiseTime"() -> (w818:dbl)
                          n228 = local read "State \"1\""() -> (w822:dbl)
                          n229 = local read "State \"0\""() -> (w821:dbl)
                          n230 = local read "FallTime"() -> (w817:dbl)
                          n231 = local read "VcMiddle"() -> (w804:string)
                          n232 = local read "VcUpper"() -> (w833:string)
                          n233 = local read "VcLower"() -> (w832:string)
                          n234 = Number To Fractional String(number=w836) -> (F-format string=w810:string)  [unwired: 3 in]
                          n235 = Number To Fractional String(number=w809) -> (F-format string=w808:string)  [unwired: 3 in]
                          n236 = Number To Fractional String(number=w806) -> (F-format string=w807:string)  [unwired: 3 in]
                          n237 = Number To Fractional String(number=w835) -> (F-format string=w834:string)  [unwired: 3 in]
                          n238 = Number To Fractional String(number=w831) -> (F-format string=w830:string)  [unwired: 3 in]
                          n239 = Number To Fractional String(number=w829) -> (F-format string=w828:string)  [unwired: 3 in]
                          n240 = Number To Fractional String(number=w826) -> (F-format string=w825:string)  [unwired: 3 in]
                          n241 = Number To Fractional String(number=w827) -> (F-format string=w824:string)  [unwired: 3 in]
                          n242 = Number To Fractional String(number=w822) -> (F-format string=w820:string)  [unwired: 3 in]
                          n243 = Number To Fractional String(number=w814) -> (F-format string=w812:string)  [unwired: 3 in]
                          n244 = Number To Fractional String(number=w821) -> (F-format string=w819:string)  [unwired: 3 in]
                          n245 = Number To Fractional String(number=w818) -> (F-format string=w816:string)  [unwired: 3 in]
                          n246 = Number To Fractional String(number=w817) -> (F-format string=w815:string)  [unwired: 3 in]
                          n247 = Concatenate Strings(w810, w805, w808, w805, w807, w805, w834, w805, w833, w805, w832, w805, w830, w805, w828, w805, w825, w805, w824, w805, "", w805, w820, w805, w819, w805, w816, w805, w815, w805, w812, w805, w811, w805, w804) -> (→"OscData":string)
                        }
                      }
                    }
                    frame #17 {
                      n248 = local read "connection information"() -> (w838:path)
                      n249 = local read "TimeStart"() -> (w839:string)
                      n250 = local read "OscData"() -> (w842:string)
                      n251 = local read "DC_SN"() -> (w841:string)
                      n252 = call "Update DatabaseO.vi"("DC_SN"=w841, "OscData"=w842, "TimeStart"=w839, "connection information"=w838) -> ()  [unwired: 8 in]
                    }
                    frame #18 {
                      n253 = Wait (ms)(milliseconds to wait=u32 500) -> ()  [unwired: 1 out]
                    }
                    frame #19 {
                      n254 = case shown="4" w845 {
                        tunnel: ["<21,0>" ("string") "<20,0>" ("string") "<19,0>" ("string") "<18,0>" ("string") "<17,0>" ("string") "<16,0>" ("string") "<15,0>" ("string") "<14,0>" ("string")] -> w847
                        frame 1, Default {
                        }
                        frame 2 {
                        }
                        frame 3 {
                        }
                        frame 4 {
                        }
                        frame 5 {
                        }
                        frame 6 {
                        }
                        frame 7 {
                        }
                        frame 8 {
                        }
                      }
                      n255 = Build Array(w847) -> (w846:string[])
                      n256 = call "Arduino Command Builder.vi"("error in"=w849, "Commands"=w846, "Arduino in"=w851) -> ("error out"=w848:errorcluster, "Arduino out"=w850:refnum<visa-resource-name>)  [unwired: 7 in]
                    }
                    frame #20 {
                      n257 = Wait (ms)(milliseconds to wait=u32 500) -> ()  [unwired: 1 out]
                    }
                  }
                }
              }
            }
          }
        }
      }
    }
    frame #4 {
      # "Turns off Saunders Temp Machine"
      n258 = Bundle(0, 6) -> (w863:cluster{i32, i32})  [unwired: 1 in]
      n259 = call "Set Temperature and Rise Time.vi"("Temperature String"="o", "Device"=w863) -> ()  [unwired: 4 in, 1 out]
    }
  }
  "error out" <- w3
  "Arduino out" <- w2
